vi "FiberSpectrograph_getEvent_largeFileObjectAvailable.vi"(8 "error in (no error)":errorcluster, 11 "logevent_largeFileObjectAvailable_Ctl":T1={"url"="", "generator"="", "version"=0.0, "byte_Size"=0, "checksum"="                                                                                                                                                                                                                                                                ", "mime_Type"="                                                                                                                                                                                                                                                                ", "id"="                                                                                                                                                                                                                                                                ", "priority"=0}) -> (0 "error out":errorcluster, 2 "function return":i32, 3 "logevent_largeFileObjectAvailable_Ctl out":T1={"url"="", "generator"="", "version"=0.0, "byte_Size"=0, "checksum"="                                                                                                                                                                                                                                                                ", "mime_Type"="                                                                                                                                                                                                                                                                ", "id"="                                                                                                                                                                                                                                                                ", "priority"=0})   [LabVIEW 2016, in "SALLV_FiberSpectrograph.lvlib"]
doc: "int FiberSpectrograph_shm_getEvent_largeFileObjectAvailableLV(FiberSpectrograph_logevent_largeFileObjectAvailableLV *logevent_largeFileObjectAvailable_Ctl );"
uses:
  SALLV_FiberSpectrograph.lvlib
  DataTypes/logevent_largeFileObjectAvailable.ctl
  SALLV_FiberSpectrograph.so
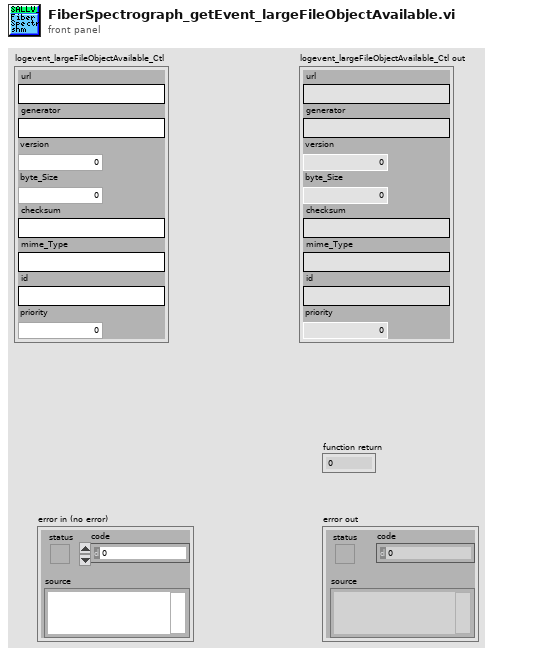
[diagram p1: front panel]
types:
  T1 = typedef "SALLV_FiberSpectrograph.lvlib/logevent_largeFileObjectAvailable.ctl" = cluster{"url":string, "generator":string, "version":sgl, "byte_Size":i32, "checksum":string, "mime_Type":string, "id":string, "priority":i32}
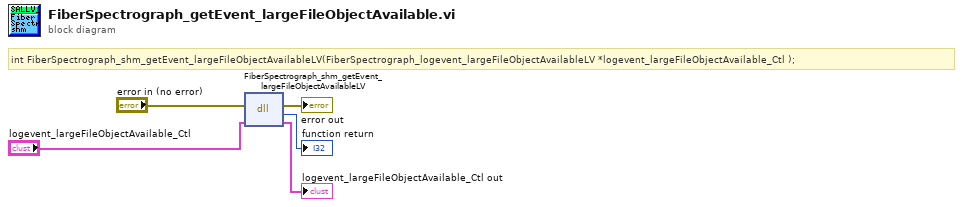
[diagram p0: block diagram]
diagram:
  # "int FiberSpectrograph_shm_getEvent_largeFileObjectAvailableLV(FiberSpectrograph_logevent_largeFileObjectAvailableLV *logevent_largeFileObjectAvailable_Ctl );"
  n1 = dll-call lib="home/harini/tcs/temp/SALLV_FiberSpectrograph.*" fn="FiberSpectrograph_shm_getEvent_largeFileObjectAvailableLV"(error in="error in (no error)", "logevent_largeFileObjectAvailable_Ctl"="logevent_largeFileObjectAvailable_Ctl") -> (error out=→"error out":errorcluster, →"function return":i32, "logevent_largeFileObjectAvailable_Ctl"=→"logevent_largeFileObjectAvailable_Ctl out":T1)  [unwired: 2 in, 1 out]
